vi "Host_STOP.vi"() -> ()   [LabVIEW 2017]
panel:
  out "ReInt Stream":bool
  in  "Master__Main.vi Refunm":refnum<vi>
  in  "cRIO Refnum":refnum<vi>
  out "Host Stop":bool
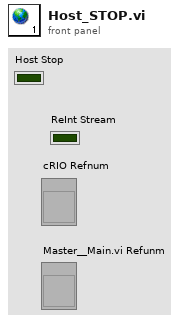
[diagram p1: front panel]
diagram:
